vi "RotateLEDs.vi"(8 "LEDs per Color":dbl=1.0, 9 "Number of LEDs":dbl, 10 "Iterations":dbl, 11 "Colors In":u32[](array[colorbox])=[16484864, 16860]) -> (3 "Colors Out":u32[](array[colorbox]))   [LabVIEW 2018]
doc: "Returns an array of colors that represents the strand of LEDs, meant to be run in a while loop and output continuously to give off a rotating effect. Colors in is an array of color objects to be used. Iterations is the while loop's current iteration. The number of LEDs is the length of the LED strand. LEDs per color is how many LEDs will be displayed in a row for each color (for example, and input array of orange and blue with an LEDs per Color of 2 will output orange, orange, blue, blue, etc.) Colors out should be put through a for loop, then get the RGB values using Color to RGB, and then assign it to the LED."
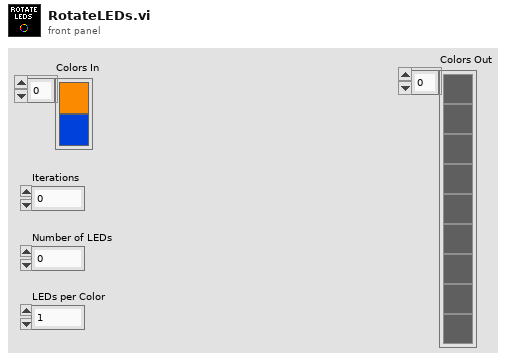
[diagram p1: front panel]
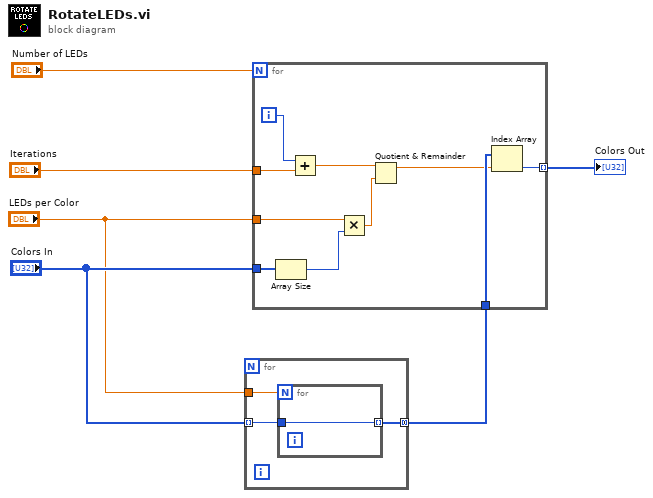
[diagram p0: block diagram]
diagram:
  n1 = for {
    tunnel: "Colors In" -> [w8] mode=indexing
    tunnel: "LEDs per Color" -> [w9]
    tunnel: [w7] -> w1 mode=concatenating
    n2 = for {
      N: w9 -> [_]
      tunnel: w8 -> [w10]
      tunnel: [w10] -> w7 mode=indexing
    }
  }
  n3 = for {
    N: "Number of LEDs" -> [_]
    tunnel: "Iterations" -> [w19]
    tunnel: [w18] -> w2 mode=indexing
    tunnel: "Colors In" -> [w17]
    tunnel: "LEDs per Color" -> [w13]
    tunnel: w1 -> [w12]
    i -> [w20]
    n4 = Array Size(array=w17) -> (size(s)=w15:i32)
    n5 = Add(x=w20, y=w19) -> (x+y=w16:dbl)
    n6 = Multiply(x=w13, y=w15) -> (x*y=w14:dbl)
    n7 = Quotient & Remainder(x=w16, y=w14) -> (x-y*floor(x/y)=w11:dbl)  [unwired: 1 out]
    n8 = Index Array(array=w12, index=w11) -> (element=w18:u32)
  }
  "Colors Out" <- w2
